vi "Convert_Always_Show_Info.vi"(7 "Array":T9[](array[typedef]) {"ERD Number" format="%.0x"}, 11 "Error In":errorcluster) -> (8 "ERD_Data_Bundled_Out":T1, 15 "Error Out":errorcluster)   [LabVIEW 2016]
doc: "This VI parses the data from ERDs in correct format, units, etc. It handles all hex to dec conversions, hex to enum, and hex to boolean conversions.\n\nIf Raw Data from ERD is blank string, then it will output values from shift register."
uses:
  Common/LabVIEW GEA2 Toolkit/LabVIEW_GEA2_Toolkit.lvlibp/type defs/ERD Read Data Out.ctl
  type defs/ERD_Data_Bundled.ctl
  type defs/ATC_Data.ctl
  type defs/Redundant.ctl
  type defs/Version.ctl
  type defs/Algorithms.ctl
  type defs/ERD_Always_Show.ctl
  type defs/Fault_Table_Info.ctl
  type defs/Cycle_Diag.ctl
  Common/LabVIEW GEA2 Toolkit/LabVIEW_GEA2_Toolkit.lvlibp
panel:
  # "Wet Load Size"
  # "Dry Load Size"
  # "OOB"
  # "Software Version"
  # "Critical Version"
  # "Non-Critical"
  # "XML Crit Ver"
  # "XML Non-Crit"
  # "Build Number"
  # "Build Hash"
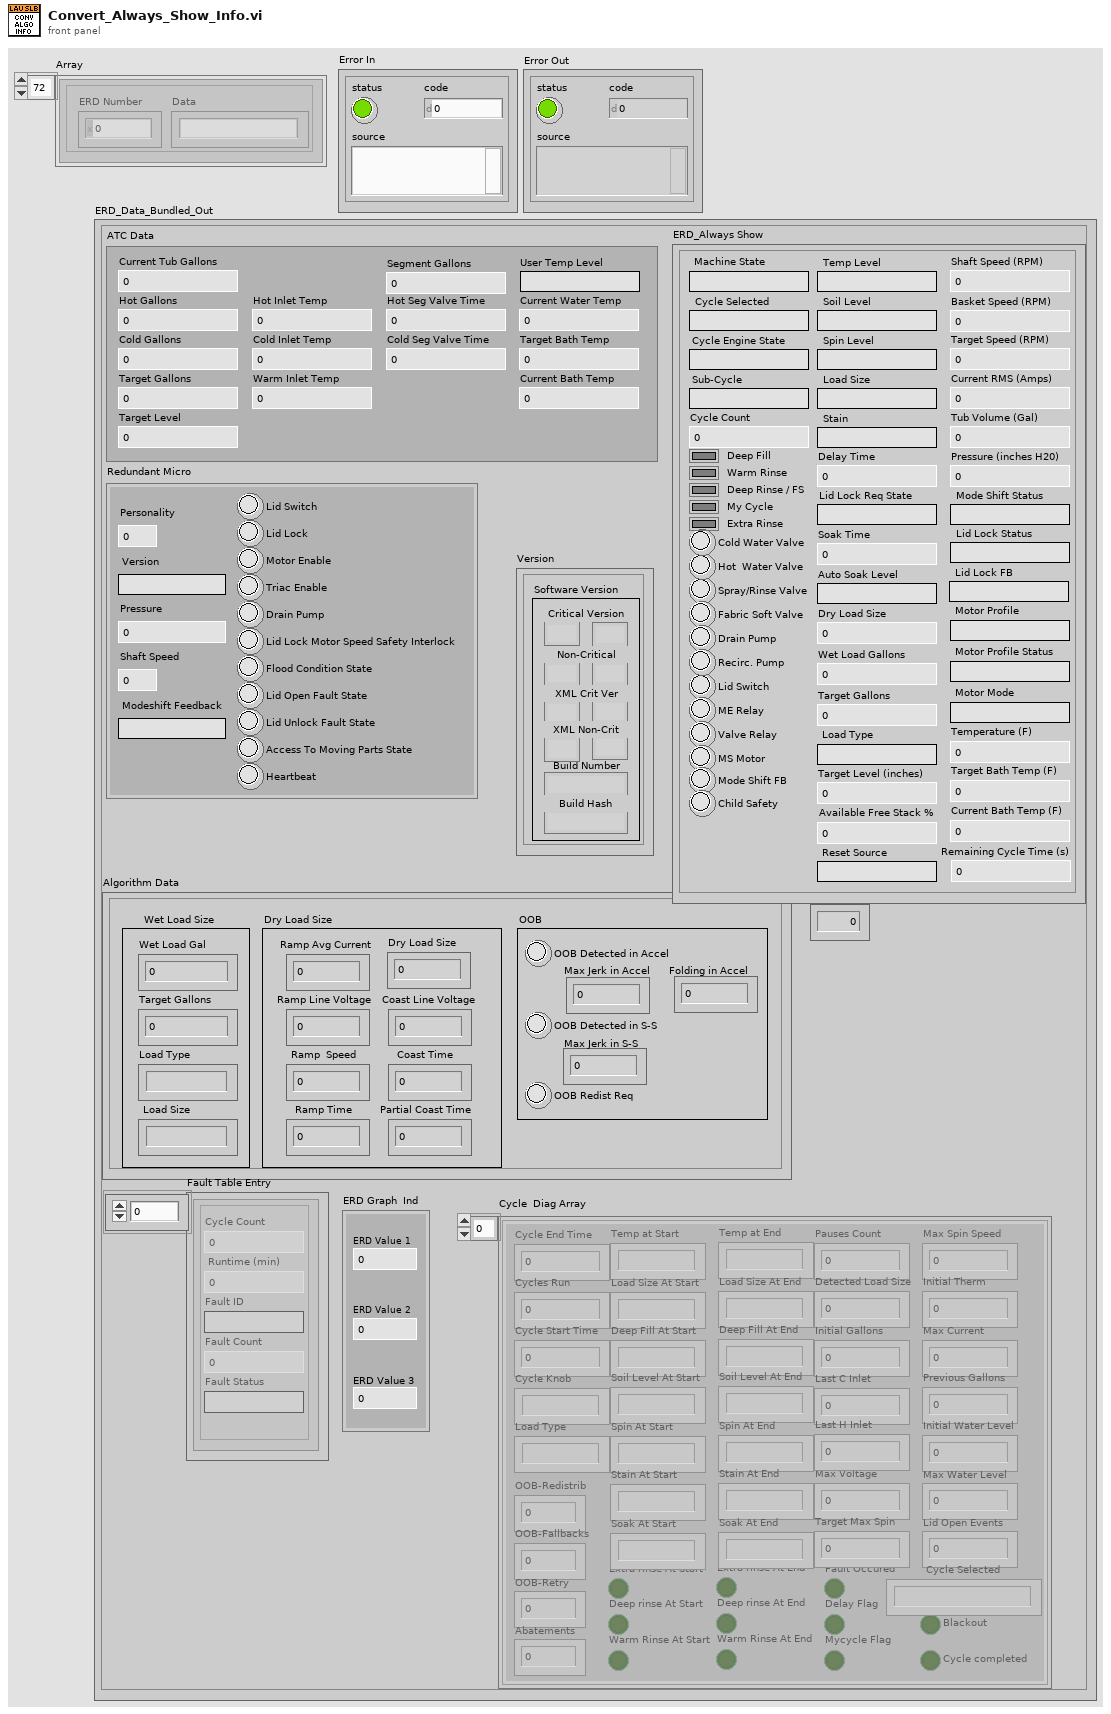
[diagram p1: front panel]
types:
  T1 = typedef "ERD_Data_Bundled.ctl" = cluster{"ATC Data":T2, "Redundant Micro":T3, "Version":T4, "Algorithm Data":T5, "ERD_Always Show":T6, "ERD Graph  Ind":cluster{"ERD Value 1":dbl, "ERD Value 2":dbl, "ERD Value 3":dbl}, "Personality Set":u8, "Fault Table Entry":T7[], "Cycle  Diag Array":T8[]}
  T2 = typedef "ATC_Data.ctl" = cluster{"Current Tub Gallons":dbl, "Hot Gallons":dbl, "Cold Gallons":dbl, "Target Gallons":dbl, "Current Water Temp":dbl, "Target Level":u32, "Target Bath Temp":dbl, "Current Bath Temp ":dbl, "Cold Inlet Temp":dbl, "Hot Inlet Temp":dbl, "Warm Inlet Temp":dbl, "Hot Seg Valve Time":u16, "Cold Seg Valve Time ":u16, "User Temp Level":string, "Segment Gallons":dbl}
  T3 = typedef "Redundant.ctl" = cluster{"Version":string, "Personality":u8, "Pressure ":dbl, "Shaft Speed":u16, "Modeshift Feedback":string, "Lid Switch":bool, "Lid Lock":bool, "Triac Enable":bool, "Drain Pump":bool, "Lid Lock Motor Speed Safety Interlock":bool, "Flood Condition State":bool, "Lid Open Fault State":bool, "Access To Moving Parts State":bool, "Heartbeat":bool, "Motor Enable":bool, "Lid Unlock Fault State":bool}
  T4 = typedef "Version.ctl" = cluster{"Critical Major":string, "Critical Minor":string, "Non-Critical Minor":string, "Non-Critical Major":string, "XML Crit Minor":string, "XMLCrit Major":string, "Build Number":string, "XML Non-crit Minor":string, "Xml Non-crit Major":string, "Build Hash":string}
  T5 = typedef "Algorithms.ctl" = cluster{"Wet Load Gal":dbl, "Target Gallons":dbl, "Load Type":string, "Load Size":string, "Coast Time":u16, "Ramp Time":u16, "Ramp  Speed":u16, "Ramp Avg Current":dbl, "OOB Redist Req":bool, "OOB Detected in S-S":bool, "Folding in Accel":i32, "Max Jerk in Accel":i32, "Max Jerk in S-S":i32, "OOB Detected in Accel":bool, "Partial Coast Time":u16, "Dry Load Size":dbl, "Ramp Line Voltage ":dbl, "Coast Line Voltage":dbl}
  T6 = typedef "ERD_Always_Show.ctl" = cluster{"Basket Speed (RPM)":u16, "Machine State":string, "Tub Volume (Gal)":dbl, "Pressure (inches H20)":dbl, "Lid Switch ":bool, "Current RMS (Amps)":dbl, "Cycle Selected":string, "Lid Lock Status":string, "Mode Shift Status":string, "Spray/Rinse Valve":bool, "Fabric Soft Valve":bool, "Drain Pump":bool, "Recirc. Pump":bool, "Cycle Engine State":string, "Hot  Water Valve":bool, "Cold Water Valve":bool, "Motor Profile":string, "Motor Profile Status":string, "Motor Mode":string, "ME Relay":bool, "Cycle Count":u32, "Deep Rinse / FS":bool, "My Cycle":bool, "Soil Level":string, "Spin Level":string, "Stain":string, "Temp Level":string, "Load Size":string, "Delay Time":u16, "Soak Time":u16, "Deep Fill":bool, "Warm Rinse":bool, "Auto Soak Level":string, "Extra Rinse":bool, "Wet Load Gallons":dbl, "Target Gallons":dbl, "Sub-Cycle":string, "Load Type":string, "Target Level (inches)":u32, "Valve Relay":bool, "Dry Load Size":dbl, "Shaft Speed (RPM) ":u16, "MS Motor":bool, "Mode Shift FB":bool, "Target Bath Temp (F)":dbl, "Temperature (F)":dbl, "Current Bath Temp (F)":dbl, "Lid Lock FB":string, "Lid Lock Req State":string, "Remaining Cycle Time (s)":u32, "Available Free Stack %":u8, "Child Safety":bool, "Target Speed (RPM)":u16, "Reset Source":string}
  T7 = typedef "Fault_Table_Info.ctl" = cluster{"Cycle Count":u32, " Runtime (min) ":u32, "Fault Status":string, "Fault ID":string, "Fault Count":u16}
  T8 = typedef "Cycle_Diag.ctl" = cluster{"Cycle End Time":u32, "Cycles Run":u32, "Cycle Start Time":u32, "Cycle Knob":string, "Load Type":string, "OOB-Redistrib":u8, "OOB-Fallbacks":u8, "OOB-Retry":u8, "Temp at Start":string, "Load Size At Start":string, "Deep Fill At Start":string, "Soil Level At Start":string, "Spin At Start":string, "Extra rinse At Start":bool, "Deep rinse At Start":bool, "Stain At Start":string, "Soak At Start":string, "Warm Rinse At Start":bool, "Temp at End":string, "Load Size At End":string, "Deep Fill At End":string, "Soil Level At End":string, "Spin At End":string, "Extra rinse At End":bool, "Deep rinse At End":bool, "Stain At End":string, "Soak At End":string, "Warm Rinse At End":bool, "Pauses Count":u8, "Fault Occured":bool, "Delay Flag":bool, "Mycycle Flag":bool, "Blackout":bool, "Cycle completed":bool, "Detected Load Size":dbl, "Initial Gallons":dbl, "Last C Inlet ":dbl, "Max Voltage":dbl, "Target Max Spin":u16, "Max Spin Speed":u16, "Initial Therm":dbl, "Max Current":dbl, "Previous Gallons":dbl, "Initial Water Level":dbl, "Max Water Level":dbl, "Abatements ":u8, "Lid Open Events":u8, "Cycle Selected":string, "Last H Inlet ":dbl}
  T9 = typedef "LabVIEW_GEA2_Toolkit.lvlibp/ERD Read Data Out.ctl" = cluster{"ERD Number":u16, "Data":string}
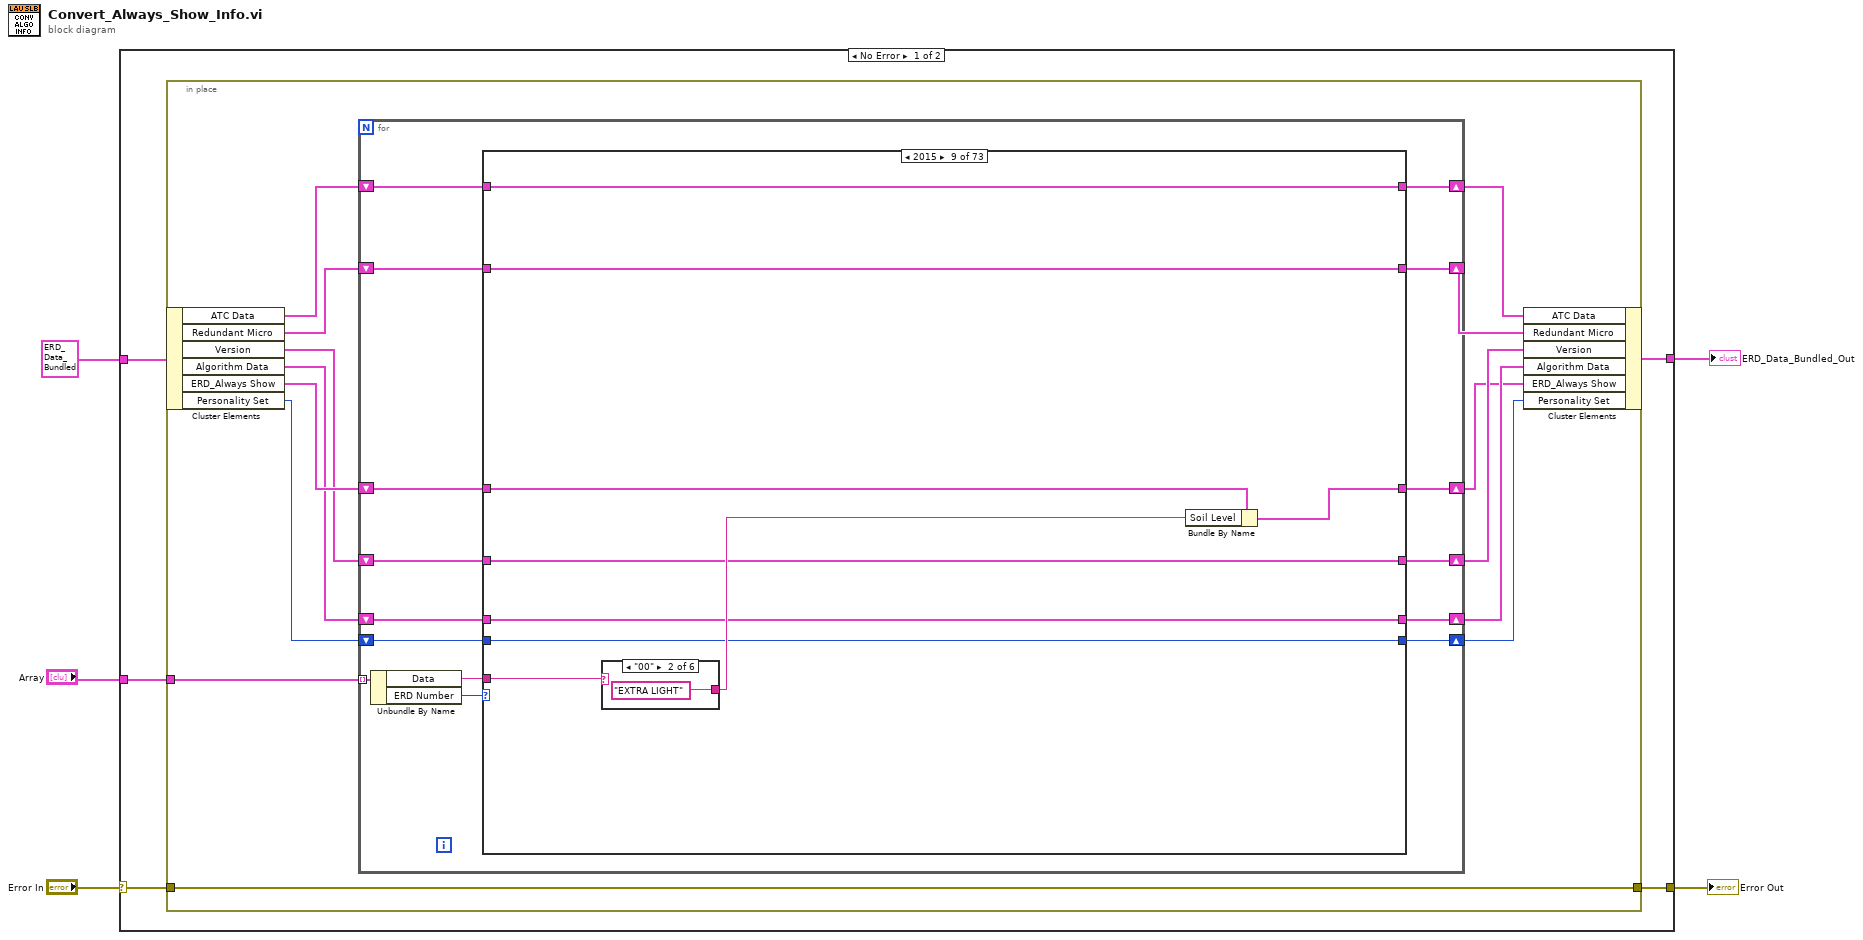
[diagram p0: block diagram]
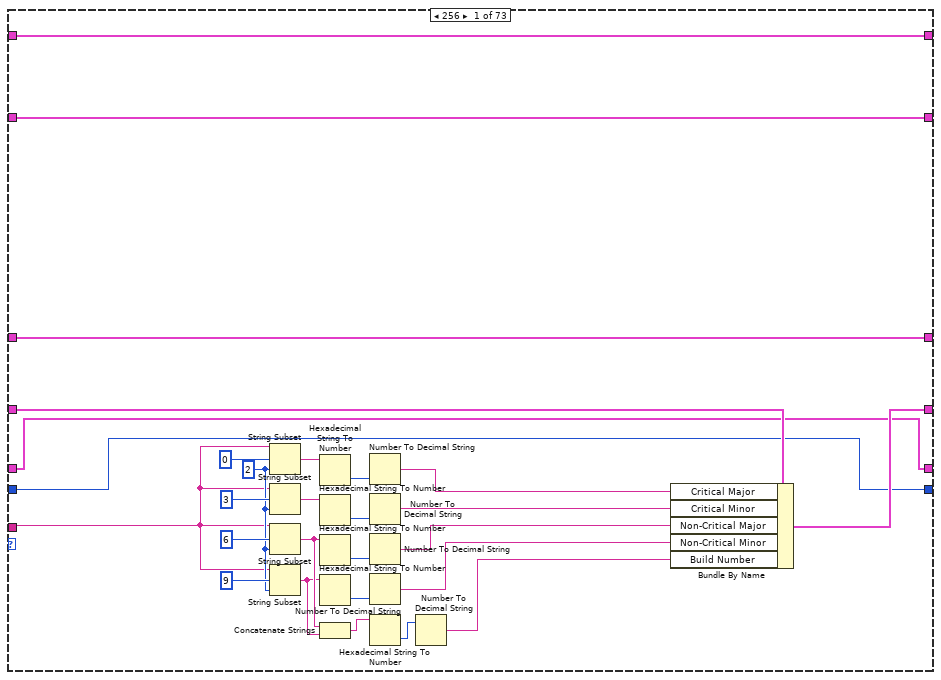
[diagram p2: hidden frame]
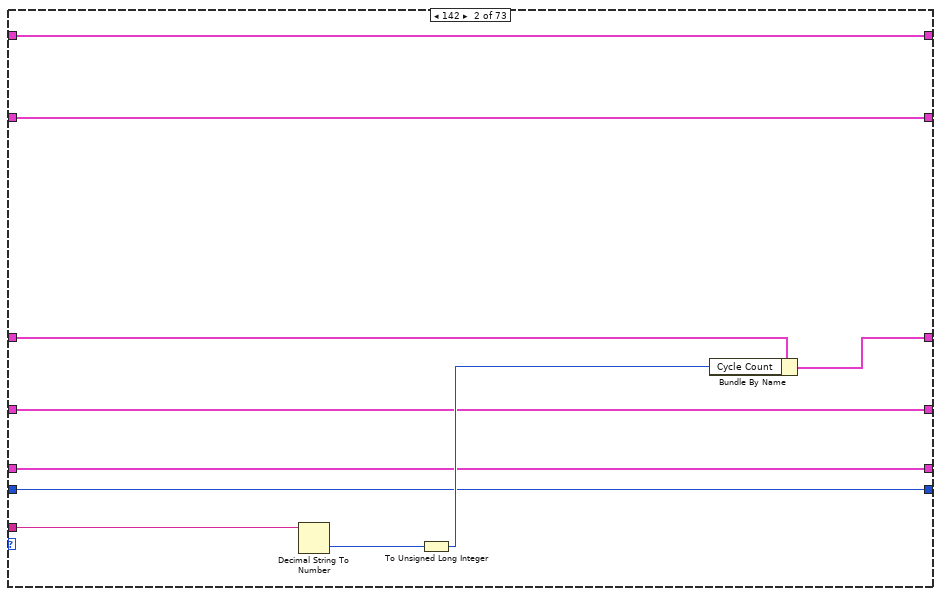
[diagram p3: hidden frame]
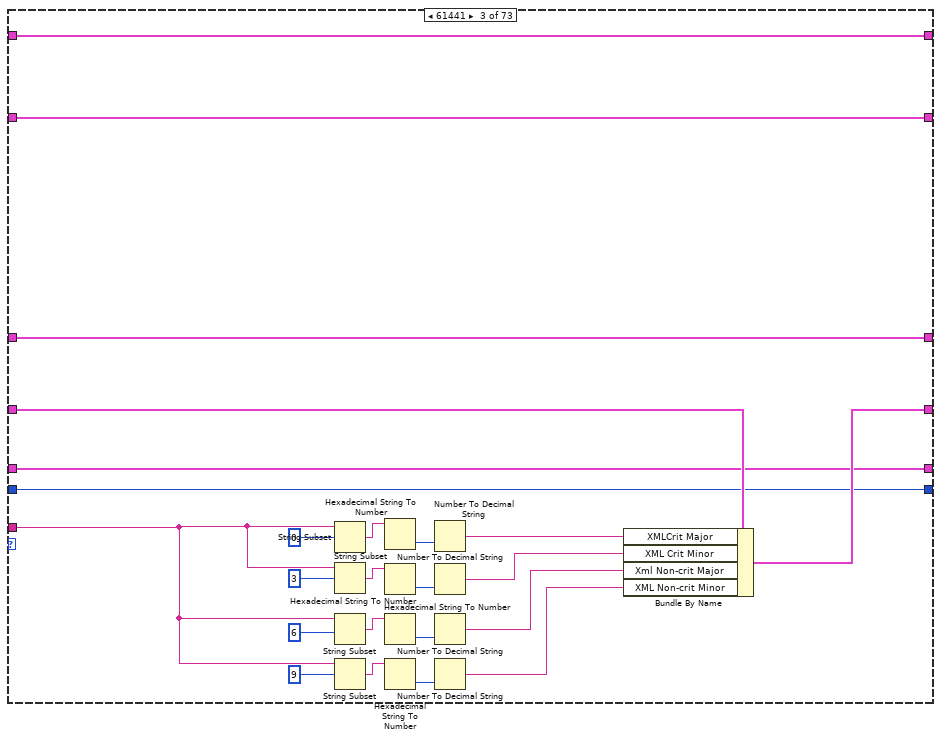
[diagram p4: hidden frame]
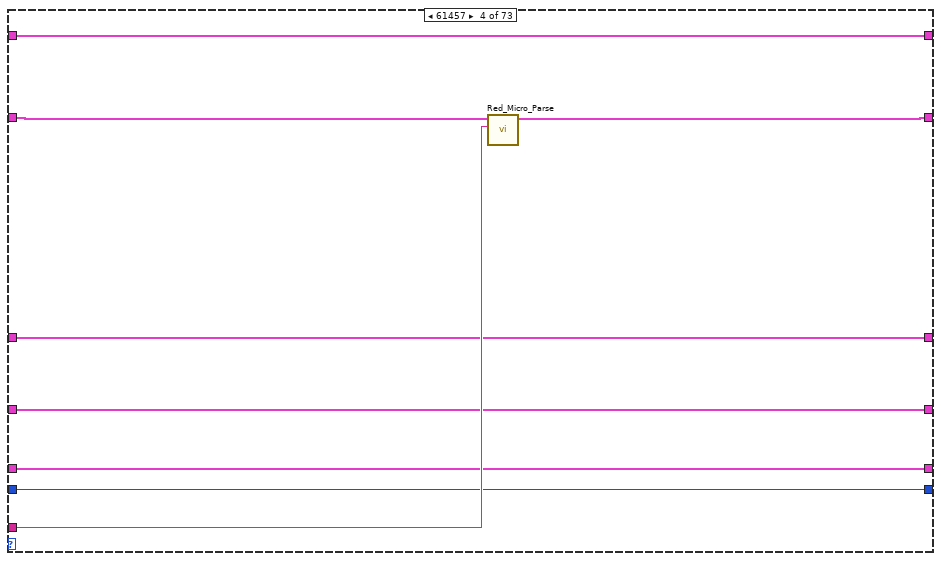
[diagram p5: hidden frame]
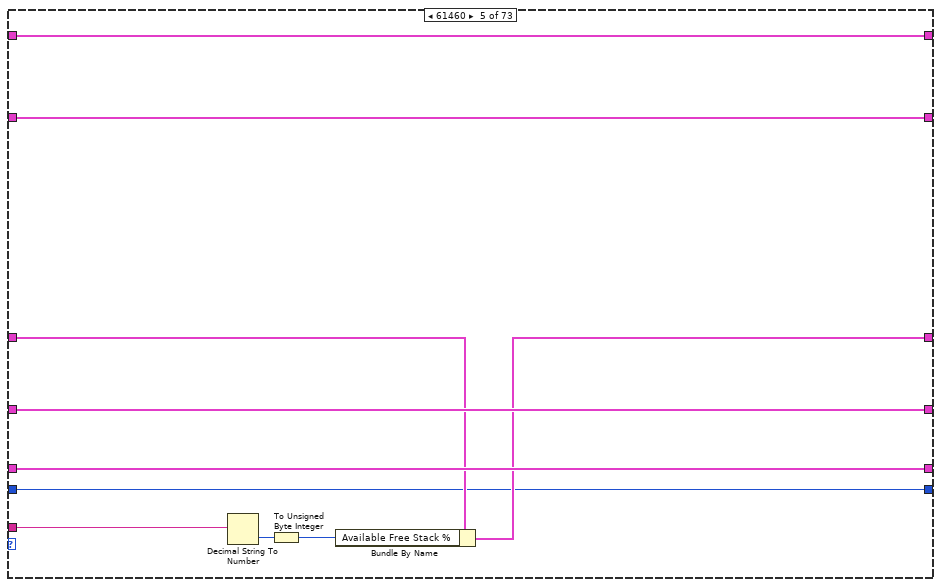
[diagram p6: hidden frame]
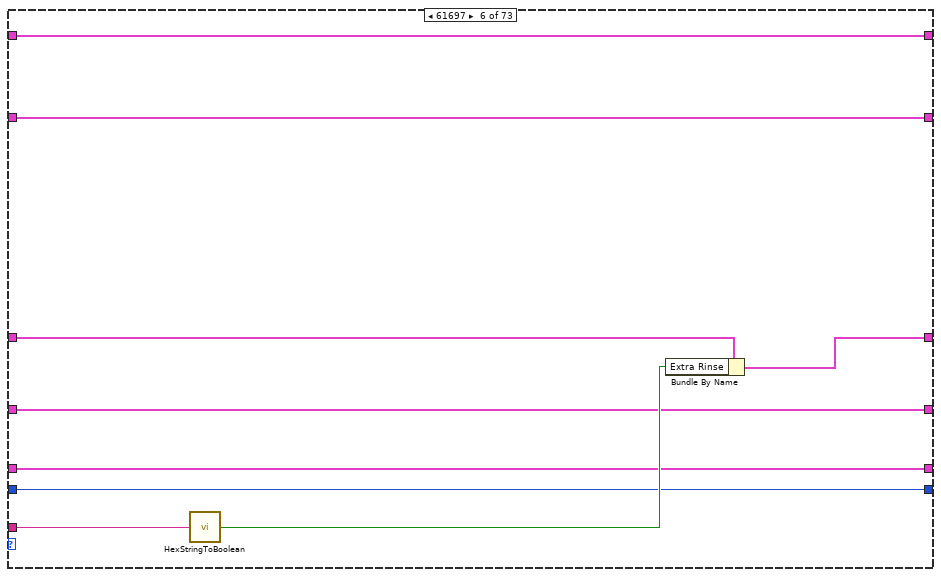
[diagram p7: hidden frame]
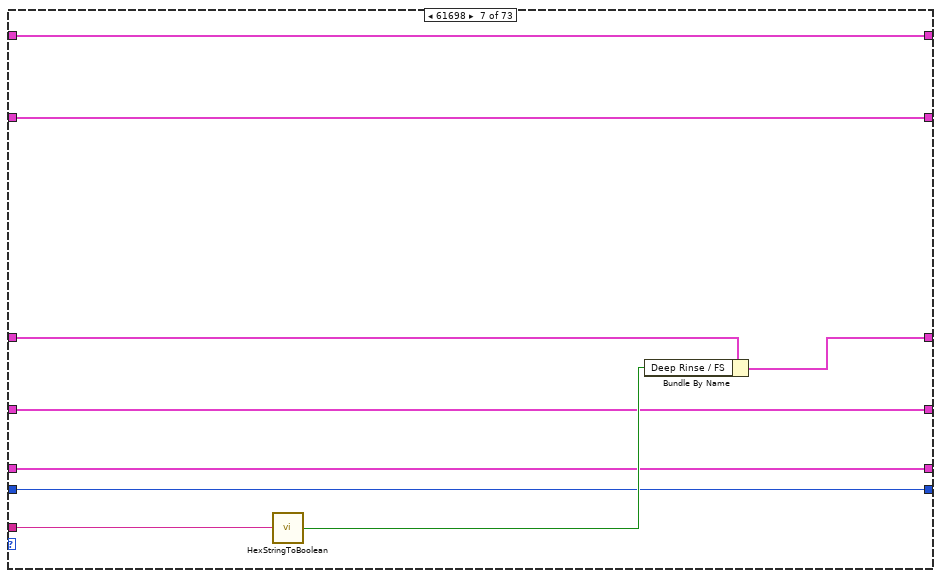
[diagram p8: hidden frame]
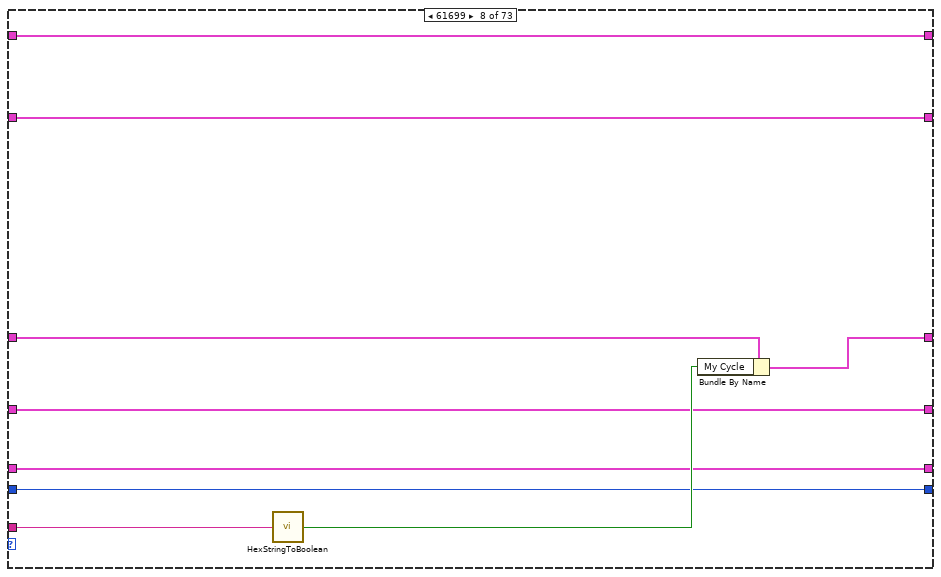
[diagram p9: hidden frame]
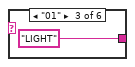
[diagram p11: hidden frame]
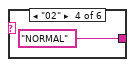
[diagram p12: hidden frame]
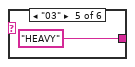
[diagram p13: hidden frame]
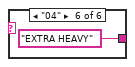
[diagram p14: hidden frame]
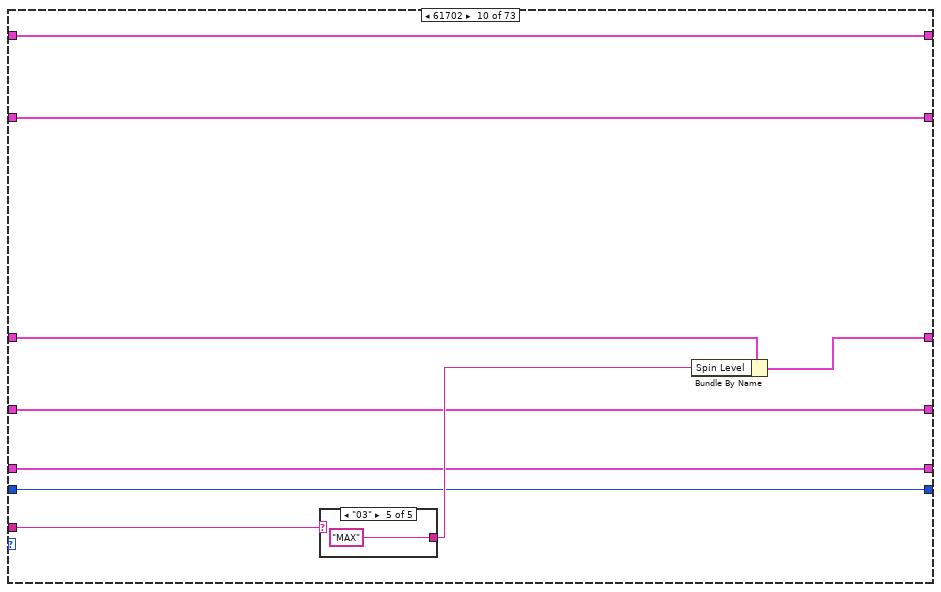
[diagram p15: hidden frame]
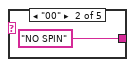
[diagram p17: hidden frame]
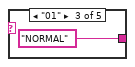
[diagram p18: hidden frame]
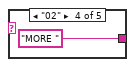
[diagram p19: hidden frame]
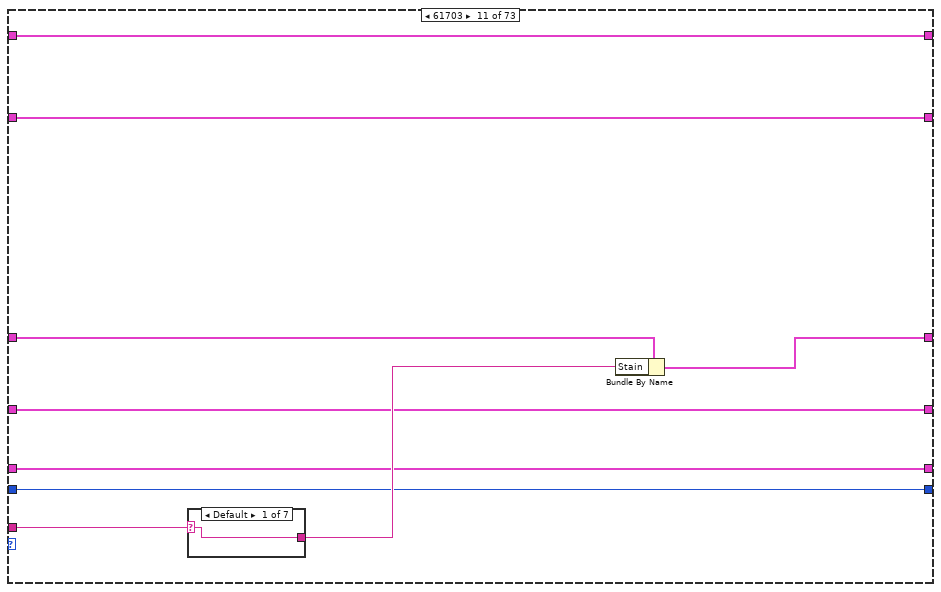
[diagram p20: hidden frame]
diagram:
  n1 = case shown="No Error" "Error In" {
    selector: "Error In" -> [w7 w1065]
    tunnel: "Array" -> [w10 _]
    tunnel: [w8 w1064] -> w3
    tunnel: T1 {"ATC Data"={"Current Tub Gallons"=0.0, "Hot Gallons"=0.0, "Cold Gallons"=0.0, "Target Gallons"=0.0, "Current Water Temp"=0.0, "Target Level"=0, "Target Bath Temp"=0.0, "Current Bath Temp "=0.0, "Cold Inlet Temp"=0.0, "Hot Inlet Temp"=0.0, "Warm Inlet Temp"=0.0, "Hot Seg Valve Time"=0, "Cold Seg Valve Time "=0, "User Temp Level"="", "Segment Gallons"=0.0}, "Redundant Micro"={"Version"="", "Personality"=0, "Pressure "=0.0, "Shaft Speed"=0, "Modeshift Feedback"="", "Lid Switch"=FALSE, "Lid Lock"=FALSE, "Triac Enable"=FALSE, "Drain Pump"=FALSE, "Lid Lock Motor Speed Safety Interlock"=FALSE, "Flood Condition State"=FALSE, "Lid Open Fault State"=FALSE, "Access To Moving Parts State"=FALSE, "Heartbeat"=FALSE, "Motor Enable"=FALSE, "Lid Unlock Fault State"=FALSE}, "Version"={"Critical Major"="", "Critical Minor"="", "Non-Critical Minor"="", "Non-Critical Major"="", "XML Crit Minor"="", "XMLCrit Major"="", "Build Number"="", "XML Non-crit Minor"="", "Xml Non-crit Major"="", "Build Hash"=""}, "Algorithm Data"={"Wet Load Gal"=0.0, "Target Gallons"=0.0, "Load Type"="", "Load Size"="", "Coast Time"=0, "Ramp Time"=0, "Ramp  Speed"=0, "Ramp Avg Current"=0.0, "OOB Redist Req"=FALSE, "OOB Detected in S-S"=FALSE, "Folding in Accel"=0, "Max Jerk in Accel"=0, "Max Jerk in S-S"=0, "OOB Detected in Accel"=FALSE, "Partial Coast Time"=0, "Dry Load Size"=0.0, "Ramp Line Voltage "=0.0, "Coast Line Voltage"=0.0}, "ERD_Always Show"={"Basket Speed (RPM)"=0, "Machine State"="", "Tub Volume (Gal)"=0.0, "Pressure (inches H20)"=0.0, "Lid Switch "=FALSE, "Current RMS (Amps)"=0.0, "Cycle Selected"="", "Lid Lock Status"="", "Mode Shift Status"="", "Spray/Rinse Valve"=FALSE, "Fabric Soft Valve"=FALSE, "Drain Pump"=FALSE, "Recirc. Pump"=FALSE, "Cycle Engine State"="", "Hot  Water Valve"=FALSE, "Cold Water Valve"=FALSE, "Motor Profile"="", "Motor Profile Status"="", "Motor Mode"="", "ME Relay"=FALSE, "Cycle Count"=0, "Deep Rinse / FS"=FALSE, "My Cycle"=FALSE, "Soil Level"="", "Spin Level"="", "Stain"="", "Temp Level"="", "Load Size"="", "Delay Time"=0, "Soak Time"=0, "Deep Fill"=FALSE, "Warm Rinse"=FALSE, "Auto Soak Level"="", "Extra Rinse"=FALSE, "Wet Load Gallons"=0.0, "Target Gallons"=0.0, "Sub-Cycle"="", "Load Type"="", "Target Level (inches)"=0, "Valve Relay"=FALSE, "Dry Load Size"=0.0, "Shaft Speed (RPM) "=0, "MS Motor"=FALSE, "Mode Shift FB"=FALSE, "Target Bath Temp (F)"=0.0, "Temperature (F)"=0.0, "Current Bath Temp (F)"=0.0, "Lid Lock FB"="", "Lid Lock Req State"="", "Remaining Cycle Time (s)"=0, "Available Free Stack %"=0, "Child Safety"=FALSE, "Target Speed (RPM)"=0, "Reset Source"=""}, "ERD Graph  Ind"={"ERD Value 1"=0.0, "ERD Value 2"=0.0, "ERD Value 3"=0.0}, "Personality Set"=0, "Fault Table Entry"=[], "Cycle  Diag Array"=[]} ("ERD_Data_Bundled_In") -> [w9 w1063]
    tunnel: [w6 w1063] -> w1
    frame No Error {
      n2 = in-place {
        in-place-border: w10 -> [w24]
        in-place-border: [w18] -> w8
        in-place-border: w7 -> [w18]
        n3 = in-place-cluster #1(w9) -> ("ATC Data"=w23:T2, "Redundant Micro"=w22:T3, "Version"=w20:T4, "Algorithm Data"=w19:T5, "ERD_Always Show"=w21:T6, "Personality Set"=w12:u8)
        n4 = for {
          tunnel: w24 -> [w39] mode=indexing
          shift-right: [w37] -> w13
          shift-left: w21 -> [w36]
          shift-right: [w34] -> w15
          shift-left: w20 -> [w35]
          shift-right: [w32] -> w16
          shift-left: w22 -> [w33]
          shift-right: [w30] -> w17
          shift-left: w23 -> [w31]
          shift-right: [w28] -> w14
          shift-left: w19 -> [w29]
          shift-right: [w25] -> w11
          shift-left: w12 -> [w26]
          n5 = Unbundle By Name(w39) -> ("Data"=w38:string, "ERD Number"=w27:u16)
          n6 = case shown="2015" w27 {
            tunnel: w38 -> [w52 w76 w88 w108 w115 w125 w136 w145 w153 w168 w181 w199 w217 w231 w248 w276 w286 w293 w298 w316 w319 w338 w351 w363 w378 w390 w411 w420 w436 w451 w463 w493 w505 w517 w527 w546 w556 w571 w584 w597 w604 w616 w628 w641 w674 w696 w710 w717 w728 w740 w750 w760 w777 w783 w806 w829 w858 w868 w877 w890 w907 w926 w935 w944 w952 w975 w989 w1001 w1010 w1013 w1023 w1034 w1048]
            tunnel: [w43 w74 w81 w106 w112 w127 w134 w143 w154 w169 w183 w200 w216 w234 w250 w274 w284 w294 w303 w314 w328 w336 w349 w360 w375 w388 w409 w423 w430 w449 w475 w491 w503 w515 w526 w544 w558 w569 w582 w595 w609 w621 w633 w665 w691 w694 w709 w721 w733 w743 w753 w765 w775 w802 w825 w848 w856 w864 w880 w885 w909 w924 w933 w942 w961 w977 w991 w999 w1007 w1016 w1028 w1040 w1043] -> w37
            tunnel: w36 -> [w43 w75 w81 w106 w114 w128 w135 w146 w155 w170 w184 w201 w218 w233 w249 w275 w285 w295 w304 w315 w318 w337 w350 w362 w376 w389 w412 w424 w432 w450 w476 w492 w504 w516 w529 w545 w559 w570 w583 w596 w609 w621 w633 w665 w691 w697 w709 w721 w733 w743 w753 w765 w776 w802 w825 w848 w857 w867 w881 w887 w910 w924 w933 w942 w960 w978 w992 w1000 w1009 w1016 w1028 w1040 w1044]
            tunnel: w35 -> [w51 w71 w89 w105 w117 w123 w132 w141 w150 w165 w179 w197 w214 w228 w246 w271 w281 w291 w301 w311 w327 w334 w347 w358 w373 w386 w408 w418 w433 w447 w460 w489 w500 w512 w524 w542 w554 w566 w580 w593 w608 w620 w632 w664 w690 w699 w707 w720 w732 w742 w752 w764 w773 w803 w826 w849 w853 w865 w874 w888 w904 w925 w934 w943 w948 w973 w987 w996 w1005 w1015 w1027 w1039 w1062]
            tunnel: [w45 w71 w83 w105 w117 w123 w132 w141 w150 w165 w179 w197 w214 w228 w246 w271 w281 w291 w301 w311 w327 w334 w347 w358 w373 w386 w408 w418 w433 w447 w460 w489 w500 w512 w524 w542 w554 w566 w580 w593 w608 w620 w632 w664 w690 w699 w707 w720 w732 w742 w752 w764 w773 w803 w826 w849 w853 w865 w874 w888 w904 w925 w934 w943 w948 w973 w987 w996 w1005 w1015 w1027 w1039 w1062] -> w34
            tunnel: w33 -> [w44 w72 w82 w109 w118 w124 w133 w142 w151 w166 w180 w198 w215 w229 w247 w272 w282 w292 w302 w312 w321 w335 w348 w359 w374 w387 w407 w419 w429 w448 w461 w490 w501 w513 w525 w543 w555 w567 w581 w594 w612 w624 w636 w666 w692 w700 w708 w722 w734 w744 w754 w766 w774 w801 w824 w847 w854 w866 w875 w884 w905 w923 w932 w941 w949 w974 w988 w997 w1006 w1017 w1029 w1038 w1061]
            tunnel: [w44 w72 w82 w107 w118 w124 w133 w142 w151 w166 w180 w198 w215 w229 w247 w272 w282 w292 w302 w312 w321 w335 w348 w359 w374 w387 w407 w419 w429 w448 w461 w490 w501 w513 w525 w543 w555 w567 w581 w594 w612 w624 w636 w666 w692 w700 w708 w722 w734 w744 w754 w766 w774 w801 w824 w847 w854 w866 w875 w884 w905 w923 w932 w941 w949 w974 w988 w997 w1006 w1017 w1029 w1038 w1061] -> w32
            tunnel: w31 -> [w42 w70 w80 w104 w119 w122 w131 w140 w149 w164 w178 w196 w213 w227 w245 w270 w280 w290 w300 w310 w320 w333 w346 w357 w372 w385 w406 w417 w428 w446 w459 w488 w499 w511 w523 w541 w553 w565 w579 w592 w611 w623 w635 w653 w682 w701 w705 w723 w735 w745 w755 w767 w772 w800 w823 w846 w852 w863 w873 w883 w903 w922 w931 w940 w947 w972 w986 w995 w1004 w1018 w1030 w1037 w1060]
            tunnel: [w42 w70 w80 w104 w119 w122 w131 w140 w149 w164 w178 w195 w213 w227 w245 w270 w280 w290 w300 w310 w320 w333 w345 w357 w371 w385 w406 w417 w428 w446 w459 w487 w499 w511 w523 w540 w553 w565 w578 w591 w610 w622 w634 w639 w673 w701 w704 w723 w735 w745 w755 w767 w772 w800 w823 w846 w852 w863 w873 w883 w903 w922 w931 w940 w947 w972 w986 w995 w1004 w1018 w1030 w1037 w1060] -> w30
            tunnel: w29 -> [w41 w69 w79 w103 w116 w121 w130 w139 w148 w163 w177 w193 w212 w226 w244 w269 w279 w289 w299 w309 w326 w332 w343 w356 w370 w384 w405 w416 w434 w445 w458 w485 w498 w510 w522 w538 w552 w564 w576 w589 w602 w614 w626 w638 w668 w698 w706 w725 w737 w747 w757 w763 w771 w799 w822 w845 w851 w862 w872 w889 w902 w921 w930 w939 w946 w971 w985 w994 w1003 w1020 w1032 w1036 w1059]
            tunnel: [w41 w69 w79 w103 w116 w121 w130 w139 w148 w163 w177 w193 w211 w226 w244 w269 w279 w289 w299 w309 w326 w331 w343 w356 w369 w383 w405 w416 w434 w445 w458 w485 w498 w510 w522 w538 w552 w564 w576 w589 w602 w614 w626 w638 w668 w698 w706 w724 w736 w746 w756 w762 w770 w798 w821 w844 w851 w862 w872 w889 w902 w920 w929 w938 w946 w971 w985 w994 w1003 w1019 w1031 w1036 w1059] -> w28
            tunnel: w26 -> [w40 w68 w78 w102 w110 w120 w129 w138 w147 w162 w176 w192 w209 w225 w242 w268 w278 w288 w296 w308 w317 w329 w342 w355 w367 w381 w404 w413 w427 w443 w456 w484 w497 w509 w521 w537 w551 w563 w575 w588 w601 w613 w625 w637 w667 w693 w702 w714 w726 w738 w748 w758 w768 w781 w804 w827 w850 w860 w870 w882 w901 w918 w927 w936 w945 w969 w984 w993 w1002 w1011 w1021 _ w1058]
            tunnel: [w40 w68 w78 w102 w110 w120 w129 w138 w147 w162 w176 w192 w209 w225 w242 w268 w278 w288 w296 w308 w317 w329 w342 w355 w367 w381 w404 w413 w427 w443 w456 w484 w497 w509 w521 w537 w551 w563 w575 w588 w601 w613 w625 w637 w667 w693 w702 w714 w726 w738 w748 w758 w768 w781 w804 w827 w850 w860 w870 w882 w901 w918 w927 w936 w945 w969 w984 w993 w1002 w1011 w1021 w1033 w1058] -> w25
            frame 256 {
              w53 = 2 ("length (rest)")
              n7 = String Subset(string=w52, offset (0)=0 ("length (rest)"), length (rest)=w53) -> (substring=w67:string)
              n8 = String Subset(string=w52, offset (0)=3 ("length (rest)"), length (rest)=w53) -> (substring=w63:string)
              n9 = String Subset(string=w52, offset (0)=6 ("length (rest)"), length (rest)=w53) -> (substring=w58:string)
              n10 = String Subset(string=w52, offset (0)=9 ("length (rest)"), length (rest)=w53) -> (substring=w57:string)
              n11 = Hexadecimal String To Number(string=w67) -> (number=w62:u32)  [unwired: 2 in, 1 out]
              n12 = Hexadecimal String To Number(string=w63) -> (number=w61:u32)  [unwired: 2 in, 1 out]
              n13 = Hexadecimal String To Number(string=w58) -> (number=w60:u32)  [unwired: 2 in, 1 out]
              n14 = Hexadecimal String To Number(string=w57) -> (number=w59:u32)  [unwired: 2 in, 1 out]
              n15 = Concatenate Strings(w58, w57) -> (w56:string)
              n16 = Number To Decimal String(number=w62) -> (decimal integer string=w50:string)  [unwired: 1 in]
              n17 = Number To Decimal String(number=w61) -> (decimal integer string=w49:string)  [unwired: 1 in]
              n18 = Number To Decimal String(number=w60) -> (decimal integer string=w48:string)  [unwired: 1 in]
              n19 = Number To Decimal String(number=w59) -> (decimal integer string=w47:string)  [unwired: 1 in]
              n20 = Hexadecimal String To Number(string=w56) -> (number=w55:u32)  [unwired: 2 in, 1 out]
              n21 = Number To Decimal String(number=w55) -> (decimal integer string=w46:string)  [unwired: 1 in]
              n22 = Bundle By Name(cluster=w51, "Critical Major"=w50, "Critical Minor"=w49, "Non-Critical Major"=w48, "Non-Critical Minor"=w47, "Build Number"=w46) -> (w45:T4)
            }
            frame 142 {
              n23 = Decimal String To Number(string=w76) -> (number=w77:i32)  [unwired: 2 in, 1 out]
              n24 = To Unsigned Long Integer(number=w77) -> (unsigned 32bit integer=w73:u32)
              n25 = Bundle By Name(cluster=w75, "Cycle Count"=w73) -> (w74:T6)
            }
            frame 61441 {
              n26 = String Subset(string=w88, offset (0)=0 ("length (rest)")) -> (substring=w99:string)  [unwired: 1 in]
              n27 = String Subset(string=w88, offset (0)=3 ("length (rest)")) -> (substring=w98:string)  [unwired: 1 in]
              n28 = String Subset(string=w88, offset (0)=6) -> (substring=w95:string)  [unwired: 1 in]
              n29 = String Subset(string=w88, offset (0)=9) -> (substring=w94:string)  [unwired: 1 in]
              n30 = Hexadecimal String To Number(string=w99) -> (number=w97:u32)  [unwired: 2 in, 1 out]
              n31 = Hexadecimal String To Number(string=w98) -> (number=w96:u32)  [unwired: 2 in, 1 out]
              n32 = Hexadecimal String To Number(string=w95) -> (number=w93:u32)  [unwired: 2 in, 1 out]
              n33 = Hexadecimal String To Number(string=w94) -> (number=w90:u32)  [unwired: 2 in, 1 out]
              n34 = Number To Decimal String(number=w97) -> (decimal integer string=w87:string)  [unwired: 1 in]
              n35 = Number To Decimal String(number=w96) -> (decimal integer string=w86:string)  [unwired: 1 in]
              n36 = Number To Decimal String(number=w93) -> (decimal integer string=w85:string)  [unwired: 1 in]
              n37 = Number To Decimal String(number=w90) -> (decimal integer string=w84:string)  [unwired: 1 in]
              n38 = Bundle By Name(cluster=w89, "XMLCrit Major"=w87, "XML Crit Minor"=w86, "Xml Non-crit Major"=w85, "XML Non-crit Minor"=w84) -> (w83:T4)
            }
            frame 61457 {
              n39 = call "Red_Micro_Parse.vi"("Data"=w108, "Redundant Micro in"=w109) -> ("Redundant Micro out"=w107:T3)  [unwired: 9 in]
            }
            frame 61460 {
              n40 = Decimal String To Number(string=w115) -> (number=w113:i32)  [unwired: 2 in, 1 out]
              n41 = To Unsigned Byte Integer(number=w113) -> (unsigned 8bit integer=w111:u8)
              n42 = Bundle By Name(cluster=w114, "Available Free Stack %"=w111) -> (w112:T6)
            }
            frame 61697 {
              n43 = call "HexStringToBoolean.vi"("Hex String"=w125) -> ("Boolean"=w126:bool)
              n44 = Bundle By Name(cluster=w128, "Extra Rinse"=w126) -> (w127:T6)
            }
            frame 61698 {
              n45 = call "HexStringToBoolean.vi"("Hex String"=w136) -> ("Boolean"=w137:bool)
              n46 = Bundle By Name(cluster=w135, "Deep Rinse / FS"=w137) -> (w134:T6)
            }
            frame 61699 {
              n47 = call "HexStringToBoolean.vi"("Hex String"=w145) -> ("Boolean"=w144:bool)
              n48 = Bundle By Name(cluster=w146, "My Cycle"=w144) -> (w143:T6)
            }
            frame 8213 {
              n49 = case shown="\"00\"" w153 {
                selector: w153 -> [w156 _ _ _ _ _]
                tunnel: [w156 "EXTRA LIGHT" "LIGHT" "NORMAL" "HEAVY" "EXTRA HEAVY"] -> w152
                frame Default {
                }
                frame "00" {
                }
                frame "01" {
                }
                frame "02" {
                }
                frame "03" {
                }
                frame "04" {
                }
              }
              n50 = Bundle By Name(cluster=w155, "Soil Level"=w152) -> (w154:T6)
            }
            frame 61702 {
              n51 = case shown="\"03\"" w168 {
                selector: w168 -> [w171 _ _ _ _]
                tunnel: [w171 "NO SPIN" "NORMAL" "MORE " "MAX"] -> w167
                frame Default {
                }
                frame "00" {
                }
                frame "01" {
                }
                frame "02" {
                }
                frame "03" {
                }
              }
              n52 = Bundle By Name(cluster=w170, "Spin Level"=w167) -> (w169:T6)
            }
            frame 61703 {
              n53 = case shown="Default" w181 {
                selector: w181 -> [w185 _ _ _ _ _ _]
                tunnel: [w185 "OFF" "TOMATO" "WINE" "BLOOD" "GRASS" "DIRT"] -> w182
                frame Default {
                }
                frame "00" {
                }
                frame "01" {
                }
                frame "02" {
                }
                frame "03" {
                }
                frame "04" {
                }
                frame "05" {
                }
              }
              n54 = Bundle By Name(cluster=w184, "Stain"=w182) -> (w183:T6)
            }
            frame 61704 {
              n55 = case shown="\"01\"" w199 {
                selector: w199 -> [w202 _ _ _ _ _ _]
                tunnel: [w202 "TAP COLD" "COLD" "COOL" "COLORS" "WARM" "HOT"] -> w194
                frame Default {
                }
                frame "00" {
                }
                frame "01" {
                }
                frame "02" {
                }
                frame "03" {
                }
                frame "04" {
                }
                frame "05" {
                }
              }
              n56 = Bundle By Name(cluster=w196, "User Temp Level"=w194) -> (w195:T2)
              n57 = Bundle By Name(cluster=w201, "Temp Level"=w194) -> (w200:T6)
            }
            frame 61705 {
              n58 = case shown="\"04\"" w217 {
                selector: w217 -> [w219 _ _ _ _ _]
                tunnel: [w219 "SMALL" "MEDIUM" "LARGE" "SUPER" "PRECISE FILL"] -> w210
                frame Default {
                }
                frame "00" {
                }
                frame "01" {
                }
                frame "02" {
                }
                frame "03" {
                }
                frame "04" {
                }
              }
              n59 = Bundle By Name(cluster=w212, "Load Size"=w210) -> (w211:T5)
              n60 = Bundle By Name(cluster=w218, "Load Size"=w210) -> (w216:T6)
            }
            frame 61706, Default {
              n61 = Decimal String To Number(string=w231) -> (number=w232:i32)  [unwired: 2 in, 1 out]
              n62 = case shown="1, Default" w232 {
                tunnel: ["IDLE" "STANDBY" "DELAY" "RUN" "PAUSE" "DELAY PAUSE" ("Profile Status") "EOC"] -> w230
                frame 1, Default {
                }
                frame 2 {
                }
                frame 4 {
                }
                frame 8 {
                }
                frame 16 {
                }
                frame 20 {
                }
                frame 32 {
                }
              }
              n63 = Bundle By Name(cluster=w233, "Machine State"=w230) -> (w234:T6)
            }
            frame 61708 {
              n64 = Decimal String To Number(string=w248) -> (number=w251:i32)  [unwired: 2 in, 1 out]
              n65 = case shown="0, Default" w251 {
                tunnel: ["Cycle 0" ("Motor Profile") "Cycle 1" ("Motor Profile") "Cycle 2" ("Motor Profile") "Cycle 3" ("Motor Profile") "Cycle 4" ("Motor Profile") "Cycle 5" ("Motor Profile") "Cycle 6" ("Motor Profile") "Cycle 7" ("Motor Profile") "Cycle 8" ("Motor Profile") "Cycle 9" ("Motor Profile") "Cycle 10" ("Motor Profile") "Cycle 11" ("Motor Profile") "Cycle 12" ("Motor Profile") "Cycle 13" ("Motor Profile") "Cycle 14" ("Motor Profile") "Cycle 15" ("Motor Profile")] -> w243
                frame 0, Default {
                }
                frame 1 {
                }
                frame 2 {
                }
                frame 3 {
                }
                frame 4 {
                }
                frame 5 {
                }
                frame 6 {
                }
                frame 7 {
                }
                frame 8 {
                }
                frame 9 {
                }
                frame 10 {
                }
                frame 11 {
                }
                frame 12 {
                }
                frame 13 {
                }
                frame 14 {
                }
                frame 15 {
                }
              }
              n66 = Bundle By Name(cluster=w249, "Cycle Selected"=w243) -> (w250:T6)
            }
            frame 8208 {
              n67 = Decimal String To Number(string=w276) -> (number=w277:i32)  [unwired: 2 in, 1 out]
              n68 = To Unsigned Word Integer(number=w277) -> (unsigned 16bit integer=w273:u16)
              n69 = Bundle By Name(cluster=w275, "Delay Time"=w273) -> (w274:T6)
            }
            frame 61710 {
              n70 = Decimal String To Number(string=w286) -> (number=w287:i32)  [unwired: 2 in, 1 out]
              n71 = To Unsigned Word Integer(number=w287) -> (unsigned 16bit integer=w283:u16)
              n72 = Bundle By Name(cluster=w285, "Soak Time"=w283) -> (w284:T6)
            }
            frame 61726 {
              n73 = Bundle By Name(cluster=w295, "Auto Soak Level"=w293) -> (w294:T6)
            }
            frame 61731 {
              n74 = case shown="\"00\", Default" w298 {
                tunnel: [FALSE ("Eco Wash") TRUE ("Eco Wash") TRUE ("Eco Wash")] -> w297
                frame "00", Default {
                }
                frame "01" {
                }
                frame "02" {
                }
              }
              n75 = Bundle By Name(cluster=w304, "Deep Fill"=w297) -> (w303:T6)
            }
            frame 61732 {
              n76 = call "HexStringToBoolean.vi"("Hex String"=w316) -> ("Boolean"=w313:bool)
              n77 = Bundle By Name(cluster=w315, "Warm Rinse"=w313) -> (w314:T6)
            }
            frame 61760 {
              n78 = Decimal String To Number(string=w319) -> (number=w323:i32)  [unwired: 2 in, 1 out]
              n79 = To Double Precision Float(number=w323) -> (double precision float=w324:dbl)
              n80 = Divide(x=w324, y=1.0) -> (x/y=w322:dbl)
              n81 = Bundle By Name(cluster=w318, "Remaining Cycle Time (s)"=w322) -> (w328:T6)
            }
            frame 61952 {
              n82 = Decimal String To Number(string=w338) -> (number=w341:i32)  [unwired: 2 in, 1 out]
              n83 = To Double Precision Float(number=w341) -> (double precision float=w340:dbl)
              n84 = Divide(x=w340, y=100.0) -> (x/y=w330:dbl)
              n85 = Bundle By Name(cluster=w332, "Wet Load Gal"=w330) -> (w331:T5)
              n86 = Bundle By Name(cluster=w337, "Wet Load Gallons"=w330) -> (w336:T6)
            }
            frame 61953 {
              n87 = Decimal String To Number(string=w351) -> (number=w352:i32)  [unwired: 2 in, 1 out]
              n88 = To Double Precision Float(number=w352) -> (double precision float=w353:dbl)
              n89 = Divide(x=w353, y=100.0) -> (x/y=w344:dbl)
              n90 = Bundle By Name(cluster=w346, "Current Tub Gallons"=w344) -> (w345:T2)
              n91 = Bundle By Name(cluster=w350, "Tub Volume (Gal)"=w344) -> (w349:T6)
            }
            frame 61954 {
              n92 = Decimal String To Number(string=w363) -> (number=w364:i32)  [unwired: 2 in, 1 out]
              n93 = To Double Precision Float(number=w364) -> (double precision float=w366:dbl)
              n94 = Divide(x=w366, y=1000.0) -> (x/y=w361:dbl)
              n95 = Bundle By Name(cluster=w362, "Pressure (inches H20)"=w361) -> (w360:T6)
            }
            frame 61957 {
              n96 = Decimal String To Number(string=w378) -> (number=w379:i32)  [unwired: 2 in, 1 out]
              n97 = To Double Precision Float(number=w379) -> (double precision float=w380:dbl)
              n98 = Divide(x=w380, y=100.0) -> (x/y=w368:dbl)
              n99 = Bundle By Name(cluster=w372, "Target Gallons"=w368) -> (w371:T2)
              n100 = Bundle By Name(cluster=w376, "Target Gallons"=w368) -> (w375:T6)
              n101 = Bundle By Name(cluster=w370, "Target Gallons"=w368) -> (w369:T5)
            }
            frame 61958 {
              n102 = case shown="\"11\"" w390 {
                selector: w390 -> [w391 _ _ _ _ _ _ _ _ _ _ _ _]
                tunnel: [w391 "UNKNOWN" "COTTON" "SYNTHETIC" "MIXED" "WET" "LOW FLOW" "SMALL" "MEDIUM" "LARGE" "SUPER" "SUPER PLUS" "MAX"] -> w382
                frame Default {
                }
                frame "0" {
                }
                frame "1" {
                }
                frame "2" {
                }
                frame "3" {
                }
                frame "4" {
                }
                frame "5" {
                }
                frame "6" {
                }
                frame "7" {
                }
                frame "8" {
                }
                frame "9" {
                }
                frame "10" {
                }
                frame "11" {
                }
              }
              n103 = Bundle By Name(cluster=w384, "Load Type"=w382) -> (w383:T5)
              n104 = Bundle By Name(cluster=w389, "Load Type"=w382) -> (w388:T6)
            }
            frame 61959 {
              n105 = call "HexStringToBoolean.vi"("Hex String"=w411) -> ("Boolean"=w410:bool)
              n106 = Bundle By Name(cluster=w412, "Lid Switch"=w410) -> (w409:T6)
            }
            frame 61961 {
              n107 = Decimal String To Number(string=w420) -> (number=w425:i32)  [unwired: 2 in, 1 out]
              n108 = Number To Boolean Array(number=w425) -> (Boolean array=w426:bool[])
              n109 = Index Array(array=w426) -> (element #1=w422:bool, element #2=w421:bool, element #3=w415:bool, element #4=w414:bool)  [unwired: 4 in]
              n110 = Bundle By Name(cluster=w424, "Hot  Water Valve"=w422, "Cold Water Valve"=w421, "Spray/Rinse Valve"=w415, "Fabric Soft Valve"=w414) -> (w423:T6)
            }
            frame 61962 {
              n111 = String Subset(string=w436, offset (0)=3, length (rest)=2 ("length (rest)")) -> (substring=w437:string)
              n112 = Hexadecimal String To Number(string=w437) -> (number=w435:u32)  [unwired: 2 in, 1 out]
              n113 = case shown="0, Default" w435 {
                tunnel: ["UNLOCKED" "LOCKED" "FAILURE"] -> w431
                frame 0, Default {
                }
                frame 1 {
                }
                frame 2 {
                }
              }
              n114 = Bundle By Name(cluster=w432, "Lid Lock Req State"=w431) -> (w430:T6)
            }
            frame 61963 {
              n115 = Decimal String To Number(string=w451) -> (number=w452:i32)  [unwired: 2 in, 1 out]
              n116 = case shown="2" w452 {
                tunnel: ["Unlocked" ("Motor Profile") "Locked" ("Motor Profile") "Failure" ("Motor Profile")] -> w444
                frame 0, Default {
                }
                frame 1 {
                }
                frame 2 {
                }
              }
              n117 = Bundle By Name(cluster=w450, "Lid Lock Status"=w444) -> (w449:T6)
            }
            frame 61964 {
              n118 = String Subset(string=w463, offset (0)=3, length (rest)=2 ("length (rest)")) -> (substring=w467:string)
              n119 = String Subset(string=w463, offset (0)=0, length (rest)=2 ("length (rest)")) -> (substring=w470:string)
              n120 = Hexadecimal String To Number(string=w470) -> (number=w469:u32)  [unwired: 2 in, 1 out]
              n121 = Hexadecimal String To Number(string=w467) -> (number=w465:u32)  [unwired: 2 in, 1 out]
              n122 = case shown="0, Default" w465 {
                tunnel: ["Unknown" "Started" "Stopped" "Paused" "Resumed" "Selected" "Completed"] -> w466
                frame 0, Default {
                }
                frame 6 {
                }
                frame 7 {
                }
                frame 8 {
                }
                frame 9 {
                }
                frame 10 {
                }
                frame 11 {
                }
              }
              n123 = Number To Decimal String(number=w469) -> (decimal integer string=w468:string)  [unwired: 1 in]
              n124 = call <vilib>:"Space Constant.vi"() -> ("String"=w464:string)
              n125 = Concatenate Strings("Cycle" ("string"), w464, w468, w464, w466) -> (w457:string)
              n126 = Bundle By Name(cluster=w476, "Cycle Engine State"=w457) -> (w475:T6)
            }
            frame 61967 {
              n127 = Decimal String To Number(string=w493) -> (number=w494:i32)  [unwired: 2 in, 1 out]
              n128 = To Double Precision Float(number=w494) -> (double precision float=w496:dbl)
              n129 = Divide(x=w496, y=10.0) -> (x/y=w486:dbl)
              n130 = Bundle By Name(cluster=w488, "Current Water Temp"=w486) -> (w487:T2)
              n131 = Bundle By Name(cluster=w492, "Temperature (F)"=w486) -> (w491:T6)
            }
            frame 61968 {
              n132 = String Subset(string=w505, offset (0)=3, length (rest)=2 ("length (rest)")) -> (substring=w506:string)
              n133 = call "HexStringToBoolean.vi"("Hex String"=w506) -> ("Boolean"=w502:bool)
              n134 = Bundle By Name(cluster=w504, "Drain Pump"=w502) -> (w503:T6)
            }
            frame 61969 {
              n135 = String Subset(string=w517, offset (0)=3, length (rest)=2 ("length (rest)")) -> (substring=w518:string)
              n136 = call "HexStringToBoolean.vi"("Hex String"=w518) -> ("Boolean"=w514:bool)
              n137 = Bundle By Name(cluster=w516, "Recirc. Pump"=w514) -> (w515:T6)
            }
            frame 61971 {
              n138 = case shown="\"00\"" w527 {
                selector: w527 -> [w530 _ _ _ _ _ _]
                tunnel: [w530 "NONE" "FILL" "SOAK" "WASH" "RINSE" "SPIN"] -> w528
                frame Default {
                }
                frame "00" {
                }
                frame "01" {
                }
                frame "02" {
                }
                frame "04" {
                }
                frame "08" {
                }
                frame "10" {
                }
              }
              n139 = Bundle By Name(cluster=w529, "Sub-Cycle"=w528) -> (w526:T6)
            }
            frame 61973 {
              n140 = Decimal String To Number(string=w546) -> (number=w550:i32)  [unwired: 2 in, 1 out]
              n141 = To Double Precision Float(number=w550) -> (double precision float=w548:dbl)
              n142 = Divide(x=w548, y=1000.0) -> (x/y=w549:dbl)
              n143 = To Unsigned Long Integer(number=w549) -> (unsigned 32bit integer=w539:u32)
              n144 = Bundle By Name(cluster=w541, "Target Level"=w539) -> (w540:T2)
              n145 = Bundle By Name(cluster=w545, "Target Level (inches)"=w539) -> (w544:T6)
            }
            frame 61976 {
              n146 = String Subset(string=w556, offset (0)=3, length (rest)=2 ("length (rest)")) -> (substring=w560:string)
              n147 = call "HexStringToBoolean.vi"("Hex String"=w560) -> ("Boolean"=w557:bool)
              n148 = Bundle By Name(cluster=w559, "Valve Relay"=w557) -> (w558:T6)
            }
            frame 61977 {
              n149 = case shown="\"01\"" w571 {
                selector: w571 -> [w572 _ _]
                tunnel: [w572 "LOCKED" ("Motor Profile") "UNLOCKED" ("Motor Profile")] -> w568
                frame "0", Default {
                }
                frame "00" {
                }
                frame "01" {
                }
              }
              n150 = Bundle By Name(cluster=w570, "Lid Lock FB"=w568) -> (w569:T6)
            }
            frame 61985 {
              (unwired) 10.0 ("y")
              n151 = Decimal String To Number(string=w584) -> (number=w587:i32)  [unwired: 2 in, 1 out]
              n152 = To Double Precision Float(number=w587) -> (double precision float=w585:dbl)
              n153 = Divide(x=w585, y=10.0) -> (x/y=w577:dbl)
              n154 = Bundle By Name(cluster=w579, "Target Bath Temp"=w577) -> (w578:T2)
              n155 = Bundle By Name(cluster=w583, "Target Bath Temp (F)"=w577) -> (w582:T6)
            }
            frame 61986 {
              n156 = Decimal String To Number(string=w597) -> (number=w598:i32)  [unwired: 2 in, 1 out]
              n157 = To Double Precision Float(number=w598) -> (double precision float=w600:dbl)
              n158 = Divide(x=w600, y=10.0) -> (x/y=w590:dbl)
              n159 = Bundle By Name(cluster=w592, "Current Bath Temp"=w590) -> (w591:T2)
              n160 = Bundle By Name(cluster=w596, "Current Bath Temp (F)"=w590) -> (w595:T6)
            }
            frame 61987 {
              n161 = Decimal String To Number(string=w604) -> (number=w605:i32)  [unwired: 2 in, 1 out]
              n162 = To Double Precision Float(number=w605) -> (double precision float=w606:dbl)
              n163 = Divide(x=w606, y=10.0) -> (x/y=w603:dbl)
              n164 = Bundle By Name(cluster=w611, "Cold Inlet Temp"=w603) -> (w610:T2)
            }
            frame 61988 {
              n165 = Decimal String To Number(string=w616) -> (number=w617:i32)  [unwired: 2 in, 1 out]
              n166 = To Double Precision Float(number=w617) -> (double precision float=w618:dbl)
              n167 = Divide(x=w618, y=10.0) -> (x/y=w615:dbl)
              n168 = Bundle By Name(cluster=w623, "Hot Inlet Temp"=w615) -> (w622:T2)
            }
            frame 61989 {
              n169 = Decimal String To Number(string=w628) -> (number=w629:i32)  [unwired: 2 in, 1 out]
              n170 = To Double Precision Float(number=w629) -> (double precision float=w630:dbl)
              n171 = Divide(x=w630, y=10.0) -> (x/y=w627:dbl)
              n172 = Bundle By Name(cluster=w635, "Warm Inlet Temp"=w627) -> (w634:T2)
            }
            frame 61990 {
              n173 = String Subset(string=w641, offset (0)=0, length (rest)=2 ("length (rest)")) -> (substring=w659:string)
              n174 = String Subset(string=w641, offset (0)=3, length (rest)=2 ("length (rest)")) -> (substring=w658:string)
              n175 = String Subset(string=w641, offset (0)=6, length (rest)=2 ("length (rest)")) -> (substring=w646:string)
              n176 = String Subset(string=w641, offset (0)=9, length (rest)=2 ("length (rest)")) -> (substring=w647:string)
              n177 = Concatenate Strings(w659, w658) -> (w657:string)
              n178 = Concatenate Strings(w646, w647) -> (w648:string)
              n179 = Hexadecimal String To Number(string=w657) -> (number=w654:u32)  [unwired: 2 in, 1 out]
              n180 = Hexadecimal String To Number(string=w648) -> (number=w651:u32)  [unwired: 2 in, 1 out]
              n181 = To Double Precision Float(number=w654) -> (double precision float=w655:dbl)
              n182 = To Double Precision Float(number=w651) -> (double precision float=w650:dbl)
              n183 = Divide(x=w655, y=100.0) -> (x/y=w652:dbl)
              n184 = Divide(x=w650, y=100.0) -> (x/y=w640:dbl)
              n185 = Bundle By Name(cluster=w653, "Hot Gallons"=w652, "Cold Gallons"=w640) -> (w639:T2)
            }
            frame 61991 {
              n186 = String Subset(string=w674, offset (0)=0, length (rest)=2 ("length (rest)")) -> (substring=w685:string)
              n187 = String Subset(string=w674, offset (0)=3, length (rest)=2 ("length (rest)")) -> (substring=w684:string)
              n188 = String Subset(string=w674, offset (0)=6, length (rest)=2 ("length (rest)")) -> (substring=w679:string)
              n189 = String Subset(string=w674, offset (0)=9, length (rest)=2 ("length (rest)")) -> (substring=w680:string)
              n190 = Concatenate Strings(w685, w684) -> (w683:string)
              n191 = Concatenate Strings(w679, w680) -> (w681:string)
              n192 = Hexadecimal String To Number(string=w683) -> (number=w672:u32)  [unwired: 2 in, 1 out]
              n193 = Hexadecimal String To Number(string=w681) -> (number=w670:u32)  [unwired: 2 in, 1 out]
              n194 = To Unsigned Word Integer(number=w672) -> (unsigned 16bit integer=w671:u16)
              n195 = To Unsigned Word Integer(number=w670) -> (unsigned 16bit integer=w669:u16)
              n196 = Bundle By Name(cluster=w682, "Hot Seg Valve Time"=w671, "Cold Seg Valve Time"=w669) -> (w673:T2)
            }
            frame 61994 {
              n197 = call "HexStringToBoolean.vi"("Hex String"=w696) -> ("Boolean"=w695:bool)
              n198 = Bundle By Name(cluster=w697, "Child Safety"=w695) -> (w694:T6)
            }
            frame 61995 {
              n199 = Decimal String To Number(string=w710) -> (number=w711:i32)  [unwired: 2 in, 1 out]
              n200 = To Double Precision Float(number=w711) -> (double precision float=w713:dbl)
              n201 = Divide(x=w713, y=100.0) -> (x/y=w703:dbl)
              n202 = Bundle By Name(cluster=w705, "Segment Gallons"=w703) -> (w704:T2)
            }
            frame 62208 {
              n203 = Decimal String To Number(string=w717) -> (number=w718:i32)  [unwired: 2 in, 1 out]
              n204 = To Double Precision Float(number=w718) -> (double precision float=w719:dbl)
              n205 = Divide(x=w719, y=1024.0) -> (x/y=w716:dbl)
              n206 = Bundle By Name(cluster=w725, "Ramp Avg Current"=w716) -> (w724:T5)
            }
            frame 62209 {
              n207 = Decimal String To Number(string=w728) -> (number=w729:i32)  [unwired: 2 in, 1 out]
              n208 = To Double Precision Float(number=w729) -> (double precision float=w730:dbl)
              n209 = Divide(x=w730, y=32.0) -> (x/y=w727:dbl)
              n210 = Bundle By Name(cluster=w737, "Coast Line Voltage"=w727) -> (w736:T5)
            }
            frame 62210 {
              n211 = Decimal String To Number(string=w740) -> (number=w741:i32)  [unwired: 2 in, 1 out]
              n212 = To Unsigned Word Integer(number=w741) -> (unsigned 16bit integer=w739:u16)
              n213 = Bundle By Name(cluster=w747, "Ramp  Speed"=w739) -> (w746:T5)
            }
            frame 62211 {
              n214 = Decimal String To Number(string=w750) -> (number=w751:i32)  [unwired: 2 in, 1 out]
              n215 = To Unsigned Word Integer(number=w751) -> (unsigned 16bit integer=w749:u16)
              n216 = Bundle By Name(cluster=w757, "Ramp Time"=w749) -> (w756:T5)
            }
            frame 62212 {
              n217 = Decimal String To Number(string=w760) -> (number=w761:i32)  [unwired: 2 in, 1 out]
              n218 = To Unsigned Word Integer(number=w761) -> (unsigned 16bit integer=w759:u16)
              n219 = Bundle By Name(cluster=w763, "Coast Time"=w759) -> (w762:T5)
            }
            frame 62213 {
              n220 = Decimal String To Number(string=w777) -> (number=w780:i32)  [unwired: 2 in, 1 out]
              n221 = To Double Precision Float(number=w780) -> (double precision float=w779:dbl)
              n222 = Divide(x=w779, y=32.0) -> (x/y=w769:dbl)
              n223 = Bundle By Name(cluster=w771, "Dry Load Size"=w769) -> (w770:T5)
              n224 = Bundle By Name(cluster=w776, "Dry Load Size"=w769) -> (w775:T6)
            }
            frame 62214 {
              n225 = String Subset(string=w783, offset (0)=0, length (rest)=2 ("length (rest)")) -> (substring=w793:string)
              n226 = String Subset(string=w783, offset (0)=3, length (rest)=2 ("length (rest)")) -> (substring=w792:string)
              n227 = String Subset(string=w783, offset (0)=6, length (rest)=2 ("length (rest)")) -> (substring=w785:string)
              n228 = String Subset(string=w783, offset (0)=9, length (rest)=2 ("length (rest)")) -> (substring=w784:string)
              n229 = Concatenate Strings(w793, w792, w785, w784) -> (w791:string)
              n230 = Hexadecimal String To Number(string=w791) -> (number=w790:u32)  [unwired: 2 in, 1 out]
              n231 = To Long Integer(number=w790) -> (32bit integer=w782:i32)
              n232 = Bundle By Name(cluster=w799, "Folding in Accel"=w782) -> (w798:T5)
            }
            frame 62215 {
              n233 = String Subset(string=w806, offset (0)=0, length (rest)=2 ("length (rest)")) -> (substring=w816:string)
              n234 = String Subset(string=w806, offset (0)=3, length (rest)=2 ("length (rest)")) -> (substring=w815:string)
              n235 = String Subset(string=w806, offset (0)=6, length (rest)=2 ("length (rest)")) -> (substring=w808:string)
              n236 = String Subset(string=w806, offset (0)=9, length (rest)=2 ("length (rest)")) -> (substring=w807:string)
              n237 = Concatenate Strings(w816, w815, w808, w807) -> (w814:string)
              n238 = Hexadecimal String To Number(string=w814) -> (number=w813:u32)  [unwired: 2 in, 1 out]
              n239 = To Long Integer(number=w813) -> (32bit integer=w805:i32)
              n240 = Bundle By Name(cluster=w822, "Max Jerk in Accel"=w805) -> (w821:T5)
            }
            frame 62216 {
              n241 = String Subset(string=w829, offset (0)=0, length (rest)=2 ("length (rest)")) -> (substring=w839:string)
              n242 = String Subset(string=w829, offset (0)=3, length (rest)=2 ("length (rest)")) -> (substring=w838:string)
              n243 = String Subset(string=w829, offset (0)=6, length (rest)=2 ("length (rest)")) -> (substring=w831:string)
              n244 = String Subset(string=w829, offset (0)=9, length (rest)=2 ("length (rest)")) -> (substring=w830:string)
              n245 = Concatenate Strings(w839, w838, w831, w830) -> (w837:string)
              n246 = Hexadecimal String To Number(string=w837) -> (number=w836:u32)  [unwired: 2 in, 1 out]
              n247 = To Long Integer(number=w836) -> (32bit integer=w828:i32)
              n248 = Bundle By Name(cluster=w845, "Max Jerk in S-S"=w828) -> (w844:T5)
            }
            frame 62218 {
              n249 = Decimal String To Number(string=w858) -> (number=w859:i32)  [unwired: 2 in, 1 out]
              n250 = To Unsigned Word Integer(number=w859) -> (unsigned 16bit integer=w855:u16)
              n251 = Bundle By Name(cluster=w857, "Shaft Speed (RPM)"=w855) -> (w856:T6)
            }
            frame 62219 {
              n252 = Decimal String To Number(string=w868) -> (number=w869:i32)  [unwired: 2 in, 1 out]
              n253 = To Unsigned Word Integer(number=w869) -> (unsigned 16bit integer=w861:u16)
              n254 = Bundle By Name(cluster=w867, "Basket Speed (RPM)"=w861) -> (w864:T6)
            }
            frame 62221 {
              n255 = Decimal String To Number(string=w877) -> (number=w878:i32)  [unwired: 2 in, 1 out]
              n256 = To Double Precision Float(number=w878) -> (double precision float=w879:dbl)
              n257 = Divide(x=w879, y=1024.0) -> (x/y=w871:dbl)
              n258 = Bundle By Name(cluster=w881, "Current RMS (Amps)"=w871) -> (w880:T6)
            }
            frame 62222 {
              n259 = String Subset(string=w890, offset (0)=0, length (rest)=2 ("length (rest)")) -> (substring=w896:string)
              n260 = String Subset(string=w890, offset (0)=3, length (rest)=2 ("length (rest)")) -> (substring=w895:string)
              n261 = Concatenate Strings(w896, w895) -> (w894:string)
              n262 = Hexadecimal String To Number(string=w894) -> (number=w893:u32)  [unwired: 2 in, 1 out]
              n263 = To Word Integer(number=w893) -> (16bit integer=w892:i16)
              n264 = Absolute Value(x=w892) -> (abs(x)=w891:i16)
              n265 = To Unsigned Word Integer(number=w891) -> (unsigned 16bit integer=w886:u16)
              n266 = Bundle By Name(cluster=w887, "Target Speed (RPM)"=w886) -> (w885:T6)
            }
            frame 62227 {
              n267 = Decimal String To Number(string=w907) -> (number=w908:i32)  [unwired: 2 in, 1 out]
              n268 = case shown="0, Default" w908 {
                tunnel: ["Closed Loop" "Closed Loop Angle" "Open Loop" "Open Loop Angle" "Coasting" "Braking" "Idle"] -> w906
                frame 0, Default {
                }
                frame 1 {
                }
                frame 2 {
                }
                frame 3 {
                }
                frame 4 {
                }
                frame 5 {
                }
                frame 6 {
                }
              }
              n269 = Bundle By Name(cluster=w910, "Motor Mode"=w906) -> (w909:T6)
            }
            frame 62229 {
              n270 = call "HexStringToBoolean.vi"("Hex String"=w926) -> ("Boolean"=w919:bool)
              n271 = Bundle By Name(cluster=w921, "OOB Detected in Accel"=w919) -> (w920:T5)
            }
            frame 62230 {
              n272 = call "HexStringToBoolean.vi"("Hex String"=w935) -> ("Boolean"=w928:bool)
              n273 = Bundle By Name(cluster=w930, "OOB Detected in S-S"=w928) -> (w929:T5)
            }
            frame 62231 {
              n274 = call "HexStringToBoolean.vi"("Hex String"=w944) -> ("Boolean"=w937:bool)
              n275 = Bundle By Name(cluster=w939, "OOB Redist Req"=w937) -> (w938:T5)
            }
            frame 62233 {
              n276 = String Subset(string=w952, offset (0)=3, length (rest)=2 ("length (rest)")) -> (substring=w957:string)
              n277 = String Subset(string=w952, offset (0)=0, length (rest)=2 ("length (rest)")) -> (substring=w954:string)
              n278 = Hexadecimal String To Number(string=w954) -> (number=w953:u32)  [unwired: 2 in, 1 out]
              n279 = case shown="\"0B\"" w957 {
                tunnel: ["Unknown" ("Profile Status") "Started" ("Profile Status") "Stopped" ("Profile Status") "Paused" ("Profile Status") "Resumed" ("Profile Status") "Selected" ("Profile Status") "Completed" ("Profile Status")] -> w951
                frame "00", Default {
                }
                frame "06" {
                }
                frame "07" {
                }
                frame "08" {
                }
                frame "09" {
                }
                frame "0A" {
                }
                frame "0B" {
                }
              }
              n280 = Number To Decimal String(number=w953) -> (decimal integer string=w950:string)  [unwired: 1 in]
              n281 = Bundle By Name(cluster=w960, "Motor Profile Status"=w951, "Motor Profile"=w950) -> (w961:T6)
            }
            frame 62237 {
              n282 = Decimal String To Number(string=w975) -> (number=w976:i32)  [unwired: 2 in, 1 out]
              n283 = case shown="4" w976 {
                tunnel: ["Unknown" ("Motor Profile") "Agitate State" ("Motor Profile") "Spin State" ("Motor Profile") "Trans to Spin" ("Motor Profile") "Trans to Agitate" ("Motor Profile")] -> w970
                frame 0, Default {
                }
                frame 1 {
                }
                frame 2 {
                }
                frame 3 {
                }
                frame 4 {
                }
              }
              n284 = Bundle By Name(cluster=w978, "Mode Shift Status"=w970) -> (w977:T6)
            }
            frame 62241 {
              n285 = call "HexStringToBoolean.vi"("Hex String"=w989) -> ("Boolean"=w990:bool)
              n286 = Bundle By Name(cluster=w992, "ME Relay"=w990) -> (w991:T6)
            }
            frame 62242 {
              n287 = call "HexStringToBoolean.vi"("Hex String"=w1001) -> ("Boolean"=w998:bool)
              n288 = Bundle By Name(cluster=w1000, "Mode Shift FB"=w998) -> (w999:T6)
            }
            frame 62243 {
              n289 = call "HexStringToBoolean.vi"("Hex String"=w1010) -> ("Boolean"=w1008:bool)
              n290 = Bundle By Name(cluster=w1009, "MS Motor"=w1008) -> (w1007:T6)
            }
            frame 62253 {
              n291 = Decimal String To Number(string=w1013) -> (number=w1014:i32)  [unwired: 2 in, 1 out]
              n292 = To Unsigned Word Integer(number=w1014) -> (unsigned 16bit integer=w1012:u16)
              n293 = Bundle By Name(cluster=w1020, "Partial Coast Time"=w1012) -> (w1019:T5)
            }
            frame 62254 {
              n294 = Decimal String To Number(string=w1023) -> (number=w1024:i32)  [unwired: 2 in, 1 out]
              n295 = To Double Precision Float(number=w1024) -> (double precision float=w1025:dbl)
              n296 = Divide(x=w1025, y=32.0) -> (x/y=w1022:dbl)
              n297 = Bundle By Name(cluster=w1032, "Ramp Line Voltage"=w1022) -> (w1031:T5)
            }
            frame 61440 {
              n298 = Decimal String To Number(string=w1034) -> (number=w1035:i32)  [unwired: 2 in, 1 out]
              n299 = To Unsigned Byte Integer(number=w1035) -> (unsigned 8bit integer=w1033:u8)
            }
            frame 61463 {
              # "Line Number"
              # "File Name CRC"
              n300 = String Subset(string=w1048, offset (0)=0, length (rest)=5 ("length (rest)")) -> (substring=w1041:string)
              n301 = String Subset(string=w1048, offset (0)=6, length (rest)=2 ("length (rest)")) -> (substring=w1053:string)
              n302 = String Subset(string=w1048, offset (0)=9, length (rest)=2 ("length (rest)")) -> (substring=w1054:string)
              n303 = Concatenate Strings(w1053, w1054) -> (w1055:string)
              n304 = Hexadecimal String To Number(string=w1055) -> (number=w1046:u32)  [unwired: 2 in, 1 out]
              n305 = Number To Decimal String(number=w1046) -> (decimal integer string=w1045:string)  [unwired: 1 in]
              n306 = call <vilib>:"Space Constant.vi"() -> ("String"=w1047:string)
              n307 = Concatenate Strings(w1041, w1047, w1045) -> (w1042:string)
              n308 = Bundle By Name(cluster=w1044, "Reset Source"=w1042) -> (w1043:T6)
            }
          }
        }
        n309 = in-place-cluster #1("ATC Data"=w17, "Redundant Micro"=w16, "Version"=w15, "Algorithm Data"=w14, "ERD_Always Show"=w13, "Personality Set"=w11) -> (w6:T1)
      }
    }
    frame Error {
      n310 = Unbundle By Name(w1065) -> ("code"=w1069:i32, "status"=w1070:bool, "source"=w1067:string)
      n311 = Equal?(x=w1069, y=-5006) -> (x = y?=w1073:bool)
      n312 = case shown="True" w1073 {
        tunnel: [w1077 FALSE] -> w1071
        tunnel: w1070 -> [w1077 _]
        tunnel: w1069 -> [w1076 w1079]
        tunnel: [w1076 w1079] -> w1068
        tunnel: [w1075 w1078] -> w1066
        tunnel: w1067 -> [w1075 w1078]
        frame False {
        }
        frame True {
        }
      }
      n313 = Bundle By Name(cluster=errorcluster {"status"=FALSE, "code"=0, "source"=""} ("error constant"), "status"=w1071, "code"=w1068, "source"=w1066) -> (w1064:errorcluster)
    }
  }
  "Error Out" <- w3
  "ERD_Data_Bundled_Out" <- w1
